vi "calculator(SubVI).vi"(9 "Y":dbl, 10 "X":dbl, 11 "Operation":enum16{"ADD", "SUBTRACT", "MULTIPLY", "DIVIDE"}(ring)) -> (3 "Numeric":dbl)   [LabVIEW 2016]
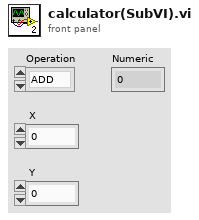
[diagram p1: front panel]
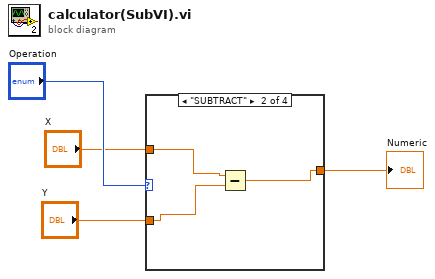
[diagram p0: block diagram]
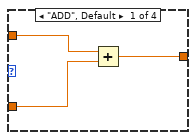
[diagram p2: hidden frame]
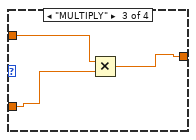
[diagram p3: hidden frame]
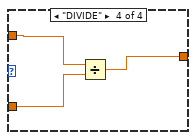
[diagram p4: hidden frame]
diagram:
  n1 = case shown="\"SUBTRACT\"" "Operation" {
    tunnel: "X" -> [w7 w10 w13 w16]
    tunnel: "Y" -> [w6 w9 w12 w15]
    tunnel: [w5 w8 w11 w14] -> w3
    frame "ADD", Default {
      n2 = Add(x=w7, y=w6) -> (x+y=w5:dbl)
    }
    frame "SUBTRACT" {
      n3 = Subtract(x=w10, y=w9) -> (x-y=w8:dbl)
    }
    frame "MULTIPLY" {
      n4 = Multiply(x=w13, y=w12) -> (x*y=w11:dbl)
    }
    frame "DIVIDE" {
      n5 = Divide(x=w16, y=w15) -> (x/y=w14:dbl)
    }
  }
  "Numeric" <- w3
